vi "Pre Launch Init.vi"(11 "TestBench in":refnum<class "TestBench.lvclass">) -> (0 "error out":errorcluster, 3 "TestBench out":refnum<class "TestBench.lvclass">)   [LabVIEW 2019, in "TestBench.lvlib" / "TestBench.lvclass"]
doc: "(<B>Filename</B>: Actor Framework.lvlib:Actor.lvclass:Pre Launch Init.vi)\n\nDefines behavior that occurs after the Launch Nested Actor method is invoked but before the actor's Actor Core method begins running.\n\nBy default, this method does nothing. A descendant class may override it to define behavior."
uses:
  TestBench.lvclass
  <vilib>/ActorFramework/Actor/Actor.lvclass
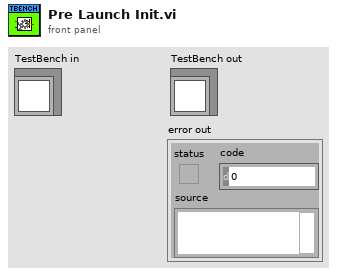
[diagram p1: front panel]
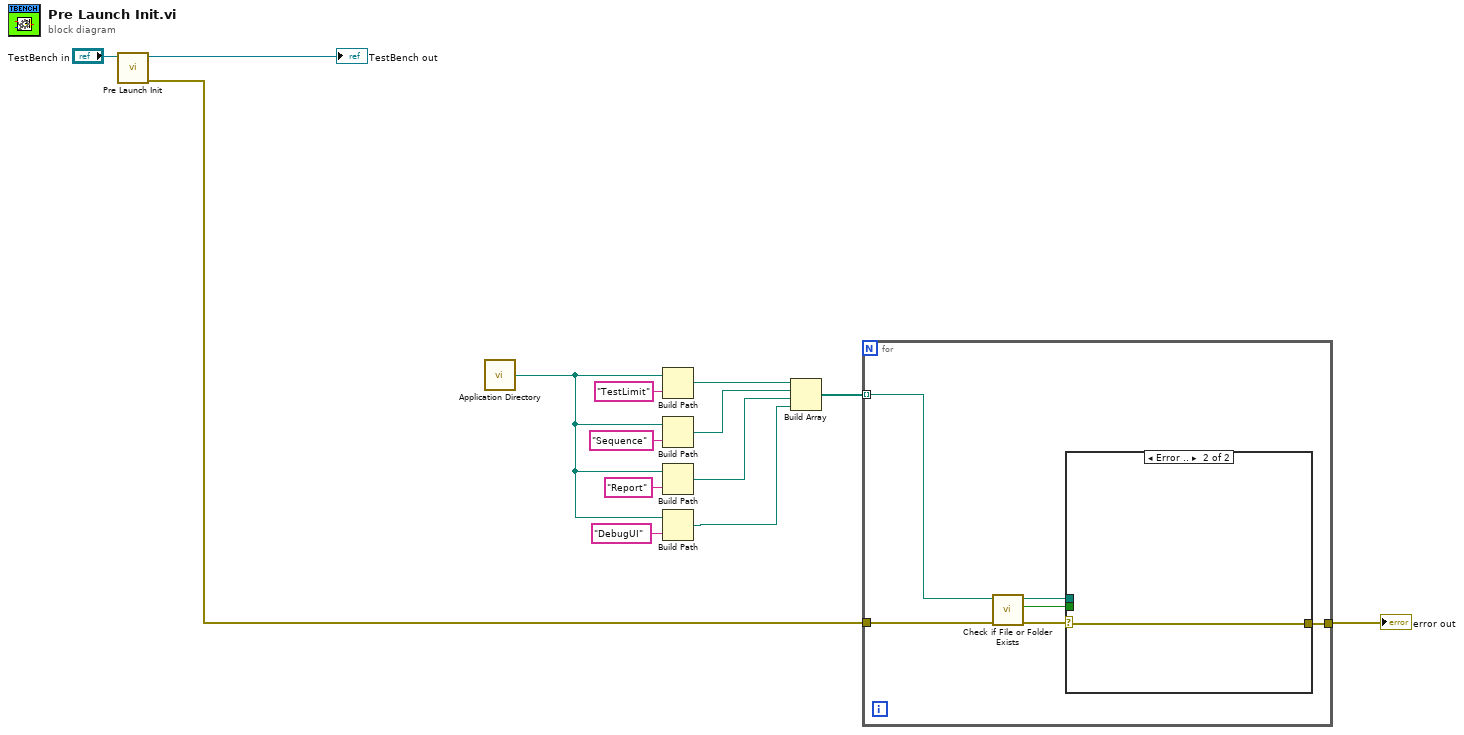
[diagram p0: block diagram]
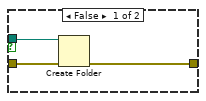
[diagram p3: hidden frame]
diagram:
  n1 = call-parent "Pre Launch Init.vi"("Actor in"="TestBench in") -> ("error out"=w2:errorcluster, "Actor out"=→"TestBench out":refnum<class "TestBench.lvclass">)  [unwired: 9 in]
  n2 = call <vilib>:"Application Directory.vi"() -> ("Application Directory"=w9:path)
  n3 = Build Path(base path=w9, name or relative path="TestLimit") -> (appended path=w7:path)
  n4 = Build Path(base path=w9, name or relative path="Sequence") -> (appended path=w6:path)
  n5 = Build Path(base path=w9, name or relative path="Report") -> (appended path=w5:path)
  n6 = Build Path(base path=w9, name or relative path="DebugUI") -> (appended path=w4:path)
  n7 = Build Array(w7, w6, w5, w4) -> (w3:path[])
  n8 = for {
    tunnel: w3 -> [w20] mode=indexing
    tunnel: w2 -> [w19]
    tunnel: [w15] -> w1
    n9 = call <vilib>:"Check if File or Folder Exists.vi"("error in (no error)"=w19, "path"=w20) -> ("error out"=w18:errorcluster, "file or folder exists?"=w17:bool, "dup path"=w16:path)  [unwired: 7 in]
    n10 = case shown="Error .." w18 {
      selector: w18 -> [w22 w29]
      tunnel: w17 -> [w24 _]
      tunnel: w16 -> [w23 _]
      tunnel: [w21 w29] -> w15
      frame No Error {
        n11 = case shown="True" w24 {
          tunnel: w23 -> [w27 _]
          tunnel: w22 -> [w26 w28]
          tunnel: [w25 w28] -> w21
          frame False {
            n12 = Create Folder(path (use dialog)=w27, error in=w26) -> (error out=w25:errorcluster)  [unwired: 1 in, 2 out]
          }
          frame True {
          }
        }
      }
      frame Error {
      }
    }
  }
  "error out" <- w1
